vi "New Gabor RefNum.vi"(7 "error in (no error)":errorcluster) -> (0 "error out":errorcluster, 3 "RefNum":T1)   [LabVIEW 2017, in "SoundVib_Gabor.lvlib"]
doc: "Creates a data block for Gabor order tracking and returns a <B>RefNum</B> referencing the data block."
uses:
  <vilib>/addons/Sound and Vibration/Order Analysis/Gabor Order Tracking/SoundVib_Gabor.lvlib
  <vilib>/addons/Sound and Vibration/Order Analysis/Ref Gabor Order Tracking/GT RefNum.ctl
  <resource>/sndvib.dll
panel:
  # "New Gabor RefNum"
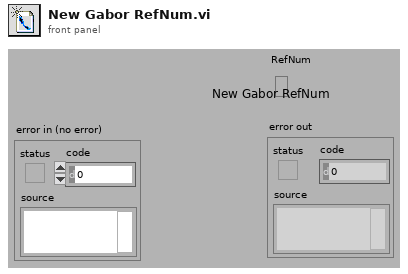
[diagram p1: front panel]
types:
  T1 = typedef "SoundVib_Gabor.lvlib/GT RefNum.ctl" = refnum<k1>
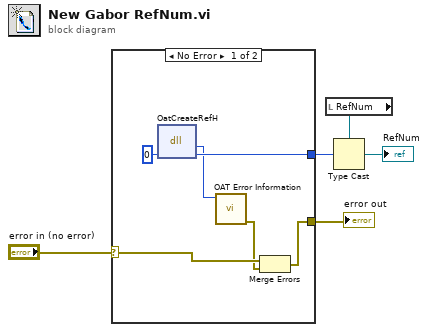
[diagram p0: block diagram]
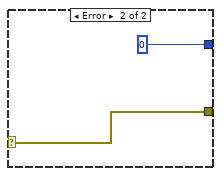
[diagram p2: hidden frame]
diagram:
  n1 = case shown="No Error" "error in (no error)" {
    selector: "error in (no error)" -> [w8 w12]
    tunnel: [w6 w12] -> w5
    tunnel: [w10 u32 0 ("GTRefNum")] -> w1
    frame No Error {
      n2 = dll-call lib="C:/Program Files (x86)/National Instruments/LabVIEW 2017/resource/sndvib.*" fn="OatCreateRefH"("GTRefNum"=u32 0) -> ("return type"=w9:i32, "GTRefNum"=w10:u32)  [unwired: 3 in, 2 out]
      n3 = call <vilib>:"OAT Error Information.vi"("error code"=w9) -> ("error out"=w7:errorcluster)  [unwired: 6 in]
      n4 = Merge Errors(w8, w7) -> (w6:errorcluster)
    }
    frame Error {
    }
  }
  "error out" <- w5
  n5 = local read "RefNum"() -> (w3:T1)
  n6 = Type Cast(type=w3, x=w1) -> (*(type *) &x=→"RefNum":T1)
